vi "_UtilsRandom2DU32Array.vi"(1 "random array size":i32=100, 2 "factor":dbl=1.0) -> (0 "random array":u32[][](array[numeric]))   [LabVIEW 2014, in "examples.lvlib"]
uses:
  examples.lvlib
  _UtilsRandomI32Array.vi
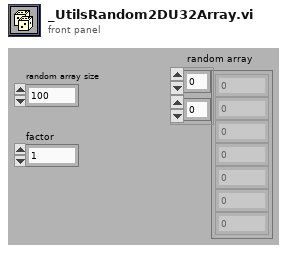
[diagram p1: front panel]
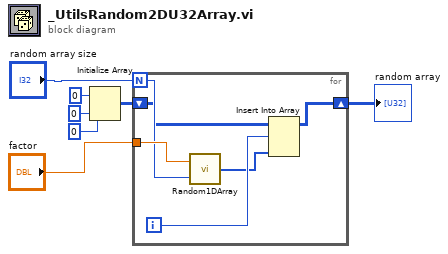
[diagram p0: block diagram]
diagram:
  n1 = Initialize Array(u32 0 ("element"), 0 ("dimension size"), 0 ("dimension size")) -> (w4:u32[][])
  n2 = for {
    N: "random array size" -> [w12]
    tunnel: "factor" -> [w13]
    shift-right: [w8] -> w3
    shift-left: w4 -> [w9]
    i -> [w11]
    n3 = call-poly "Random1DArray.vi"("array size"=w12, "factor"=w13) -> ("array"=w10:u32[])
    n4 = Insert Into Array(array=w9, index (row)=w11, new element=w10) -> (w8:u32[][])  [unwired: 1 in]
  }
  "random array" <- w3
